vi "ATF-Pump-Time Event Trigger.vi"(8 "error in":errorcluster) -> (0 "error out":errorcluster)   [LabVIEW 2022 SP3]
panel:
  out "Current time":timestamp
  in  "resource name":tag="PXI2Slot11"
  in  "Output Terminal":tag="/PXI2Slot11/PFI0"
  out "Event Time":timestamp format="%<%I:%M:%S%9u %p\n%x>T"
  in  "Start Time Delay (Seconds)":ext=5.0
  in  "Output level":enum32{"low", "high"}(ring)=enum."high"
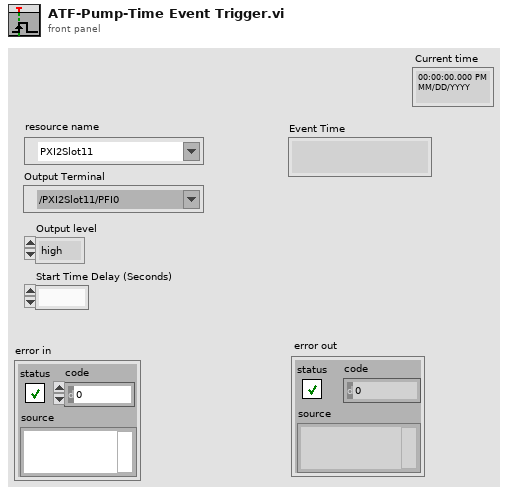
[diagram p1: front panel]
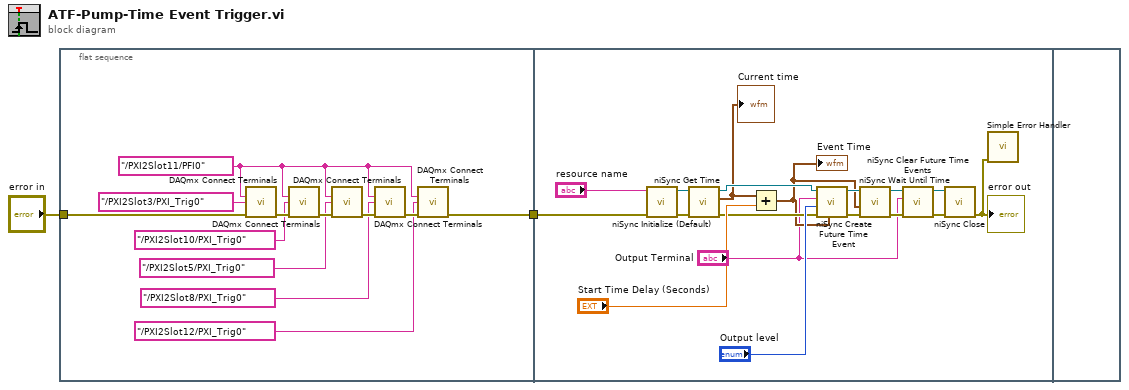
[diagram p0: block diagram]
diagram:
  n1 = flat-sequence {
    tunnel: "error in" -> [w13]
    tunnel: [w4] -> w1
    tunnel: w1 -> [w16]
    frame #0 {
      w3 = tag "/PXI2Slot11/PFI0" ("source terminal")
      n2 = call <vilib>:"DAQmx Connect Terminals.vi"("source terminal"=w3, "destination terminal"=tag "/PXI2Slot3/PXI_Trig0", "error in"=w13) -> ("error out"=w12:errorcluster)  [unwired: 12 in]
      n3 = call <vilib>:"DAQmx Connect Terminals.vi"("source terminal"=w3, "destination terminal"=tag "/PXI2Slot10/PXI_Trig0", "error in"=w12) -> ("error out"=w10:errorcluster)  [unwired: 12 in]
      n4 = call <vilib>:"DAQmx Connect Terminals.vi"("source terminal"=w3, "destination terminal"=tag "/PXI2Slot5/PXI_Trig0", "error in"=w10) -> ("error out"=w8:errorcluster)  [unwired: 12 in]
      n5 = call <vilib>:"DAQmx Connect Terminals.vi"("source terminal"=w3, "destination terminal"=tag "/PXI2Slot8/PXI_Trig0" ("source terminal"), "error in"=w8) -> ("error out"=w6:errorcluster)  [unwired: 12 in]
      n6 = call <vilib>:"DAQmx Connect Terminals.vi"("source terminal"=w3, "destination terminal"=tag "/PXI2Slot12/PXI_Trig0", "error in"=w6) -> ("error out"=w4:errorcluster)  [unwired: 12 in]
    }
    frame #1 {
      n7 = call <instrlib>:"niSync Initialize (Default).vi"("error in (no error)"=w16, "resource name"="resource name") -> ("error out"=w21:errorcluster, "instrument handle out"=w22:refnum<k15>)  [unwired: 8 in]
      n8 = call <instrlib>:"niSync Get Time.vi"("error in (no error)"=w21, "instrument handle"=w22) -> ("error out"=w28:errorcluster, "time"=w15:timestamp, "instrument handle out"=w29:refnum<k15>)  [unwired: 5 in]
      "Current time" <- w15
      n9 = Add(x=w15, y="Start Time Delay (Seconds)") -> (x+y=w25:timestamp)
      "Event Time" <- w25
      n10 = call <instrlib>:"niSync Create Future Time Event.vi"("time"=w25, "error in (no error)"=w28, "output level"="Output level", "terminal"="Output Terminal", "instrument handle"=w29) -> ("error out"=w26:errorcluster, "instrument handle out"=w27:refnum<k15>)  [unwired: 4 in]
      n11 = call <instrlib>:"niSync Wait Until Time.vi"("error in (no error)"=w26, "time stamp"=w25, "instrument handle"=w27) -> ("error out"=w24:errorcluster, "instrument handle out"=w23:refnum<k15>)  [unwired: 3 in]
      n12 = call <instrlib>:"niSync Clear Future Time Events.vi"("error in (no error)"=w24, "terminal"="Output Terminal", "instrument handle"=w23) -> ("error out"=w19:errorcluster, "instrument handle out"=w20:refnum<k15>)  [unwired: 6 in]
      n13 = call <instrlib>:"niSync Close.vi"("error in (no error)"=w19, "instrument handle"=w20) -> ("error out"=w32:errorcluster)  [unwired: 9 in]
      "error out" <- w32
      n14 = call <vilib>:"Simple Error Handler.vi"("error in (no error)"=w32) -> ()  [unwired: 4 in, 5 out]
    }
    frame #2 {
    }
  }
